vi "GetAprilTags.vi"() -> (4 "Vision Timestamp (ms)":u32, 6 "Vision Target Valid [t-?]":bool, 7 "AprilTag Data [t-?]":dbl[](array[numeric]))   [LabVIEW 2020]
doc: "Reads the raw data from the LimeLight camera assigned to detecting AprilTags. Performs some minor transformations, conducts intial validity checks, and estimates the vision data timestamp."
uses:
  2d64956e-cf35-4d84-838e-e30eff74bf58.vi
  <vilib>/Rock Robotics/Network Tables/NT Read Number.vi
  GlobalDriverStationData.vi
  <vilib>/Rock Robotics/Network Tables/NT Read Numeric Array.vi
  GlobalPoseAndTargeting.vi
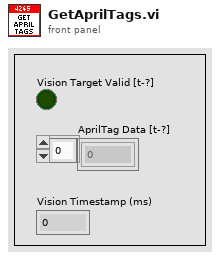
[diagram p1: front panel]
types:
  T1 = enum16{"Boot Up", "Camera Override", "HUB Targeting", "CARGO Tracking"}
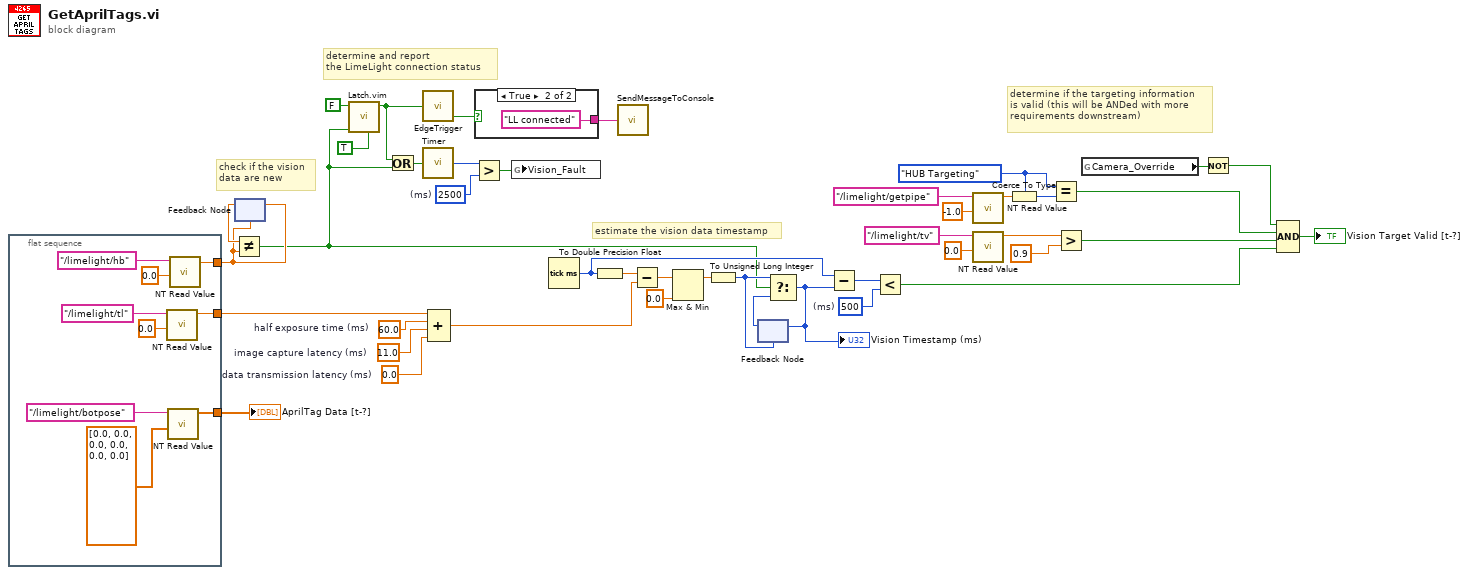
[diagram p0: block diagram]
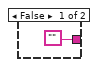
[diagram p2: hidden frame]
diagram:
  w1 = 60.0  # half exposure time (ms)
  w3 = 0.0  # data transmission latency (ms)
  w17 = u32 2500  # (ms)
  w9 = u32 500  # (ms)
  w2 = 11.0  # image capture latency (ms)
  w34 = T1."HUB Targeting" ("x")
  # "determine and report\nthe LimeLight connection status"
  # "determine if the targeting information\nis valid (this will be ANDed with more\nrequirements downstream)"
  # "estimate the vision data timestamp"
  # "check if the vision\ndata are new"
  n1 = flat-sequence {
    tunnel: [w48] -> w7
    tunnel: [w47] -> w6
    tunnel: [w44] -> w4
    frame #0 {
      n2 = call-poly <vilib>:"NT Read Value.vi"("default value"=0.0 ("Default Value"), "name"="/limelight/tl" ("Name")) -> ("value"=w48:dbl)  [unwired: 7 in, 2 out]
      n3 = call-poly <vilib>:"NT Read Value.vi"("default value"=dbl[] [0.0, 0.0, 0.0, 0.0, 0.0, 0.0], "name"="/limelight/botpose" ("Name")) -> ("value"=w44:dbl[])  [unwired: 7 in, 2 out]
      n4 = call-poly <vilib>:"NT Read Value.vi"("default value"=0.0 ("Default Value"), "name"="/limelight/hb" ("Name")) -> ("value"=w47:dbl)  [unwired: 7 in, 2 out]
    }
  }
  n5 = feedback-in #1(w6) -> ()
  n6 = feedback #1(w6) -> (w19:dbl)
  n7 = Not Equal?(x=w19, y=w6) -> (x != y?=w5:bool)
  n8 = call "Latch.vim"("Default Value"=TRUE, "Latch Signal"=w5, "Latch Value"=FALSE) -> ("Latched"=w13:bool)  [unwired: 8 in]
  n9 = Or(x=w13, y=w5) -> (x .or. y?=w16:bool)
  n10 = call "EdgeTrigger.vi"("Input Signal"=w13) -> ("Falling Edge Trigger"=w11:bool)  [unwired: 2 out]
  n11 = call "Timer.vi"("Reset Timer"=w16) -> ("Time (ms)"=w18:u32)
  n12 = Compound Arithmetic op=ADD(w7, w1, w2, w3) -> (w31:dbl)
  n13 = Greater?(x=w18, y=w17) -> (0:w8:bool)
  n14 = case shown="True" w11 {
    tunnel: ["" "LL connected" ("Message")] -> w12
    frame False {
    }
    frame True {
    }
  }
  n15 = global write "GlobalPoseAndTargeting.vi" "Vision_Fault"(w8) -> ()
  n16 = Tick Count (ms)() -> (millisecond timer value=w24:u32)
  n17 = To Double Precision Float(number=w24) -> (double precision float=w30:dbl)
  n18 = call "SendMessageToConsole.vi"("Message String"=w12) -> ()  [unwired: 1 in]
  n19 = Subtract(x=w30, y=w31) -> (x-y=w29:dbl)
  n20 = Max & Min(x=w29, y=0.0) -> (max(x,y)=w27:dbl)  [unwired: 1 out]
  n21 = To Unsigned Long Integer(number=w27) -> (unsigned 32bit integer=w26:u32)
  n22 = feedback #2(w26) -> (w32:u32)
  n23 = Select(t=w26, s=w5, f=w32) -> (s? t:f=w25:u32)
  "Vision Timestamp (ms)" <- w25
  n24 = feedback-in #2(w25) -> ()
  n25 = Subtract(x=w24, y=w25) -> (x-y=w23:u32)
  n26 = Less?(x=w23, y=w9) -> (x < y?=w22:bool)
  n27 = call-poly <vilib>:"NT Read Value.vi"("default value"=-1.0 ("Default Value"), "name"="/limelight/getpipe" ("Name")) -> ("value"=w37:dbl)  [unwired: 7 in, 2 out]
  n28 = call-poly <vilib>:"NT Read Value.vi"("default value"=0.0 ("Default Value"), "name"="/limelight/tv" ("Name")) -> ("value"=w43:dbl)  [unwired: 7 in, 2 out]
  n29 = Coerce To Type(0:w37, 1:w34) -> (2:w36:T1)
  n30 = Equal?(x=w34, y=w36) -> (x = y?=w35:bool)
  n31 = Greater?(x=w43, y=0.9) -> (0:w33:bool)
  n32 = global read "GlobalDriverStationData.vi" "Camera_Override"() -> (w21:bool)
  n33 = Not(x=w21) -> (.not. x?=w20:bool)
  n34 = Compound Arithmetic op=AND(w20, w35, w33, w22) -> (→"Vision Target Valid [t-?]":bool)
  "AprilTag Data [t-?]" <- w4
